vi "SubVI_StopDecoder.vi"(2 "error in":errorcluster, 3 "decoder in":u64) -> (0 "error":errorcluster)   [LabVIEW 2021]
uses:
  niimaqdx.dll
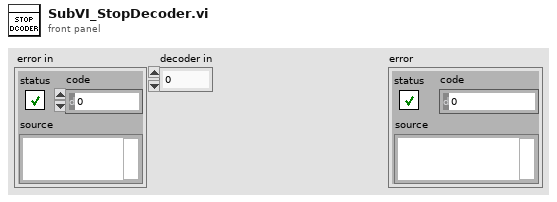
[diagram p1: front panel]
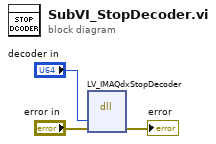
[diagram p0: block diagram]
diagram:
  n1 = dll-call lib="niimaqdx.dll" fn="LV_IMAQdxStopDecoder"("decoder"="decoder in", "error"="error in") -> ("error"=→"error":errorcluster)  [unwired: 3 in, 4 out]
